vi "EEG - Independent Component Analysis.vi"() -> ()   [LabVIEW 2013]
uses:
  <vilib>/addons/Time Series Analysis/Statistical Analysis.llb/TSA Independent Component Analysis (Waveform).vi
  <vilib>/addons/Time Series Analysis/Statistical Analysis.llb/TSA Independent Component Analysis (Array).vi
  <vilib>/addons/_Advanced Signal Processing/NI_AdvSigProcTSA.lvlib
panel:
  in  "Podesavanja za metod Fast ICA":T1={"metod"=1, "maksimalna iteracija"=1000, "tolerancija konvergencije"=1e-06, "tolerancija deflacije"=1e-14, "maksimalna preciznost"=10, "tolerancija preciznosti"=1e-08} {"metod" items=["Square", "Cube", "Tanh", "Gaussian"]}
  out "Graficki prikaz rezultata":waveform(dbl)[](graph)
  out "Lokacija sacuvanog fajla na racunaru":path
  out "Signal pre analize":waveform(dbl)[](graph)
  in  "Broj nezavisnih komponenti":i32=-1
  in  "ICA metod":u16(ring) items=["Matrix Pencil ICA", "Fast ICA"]
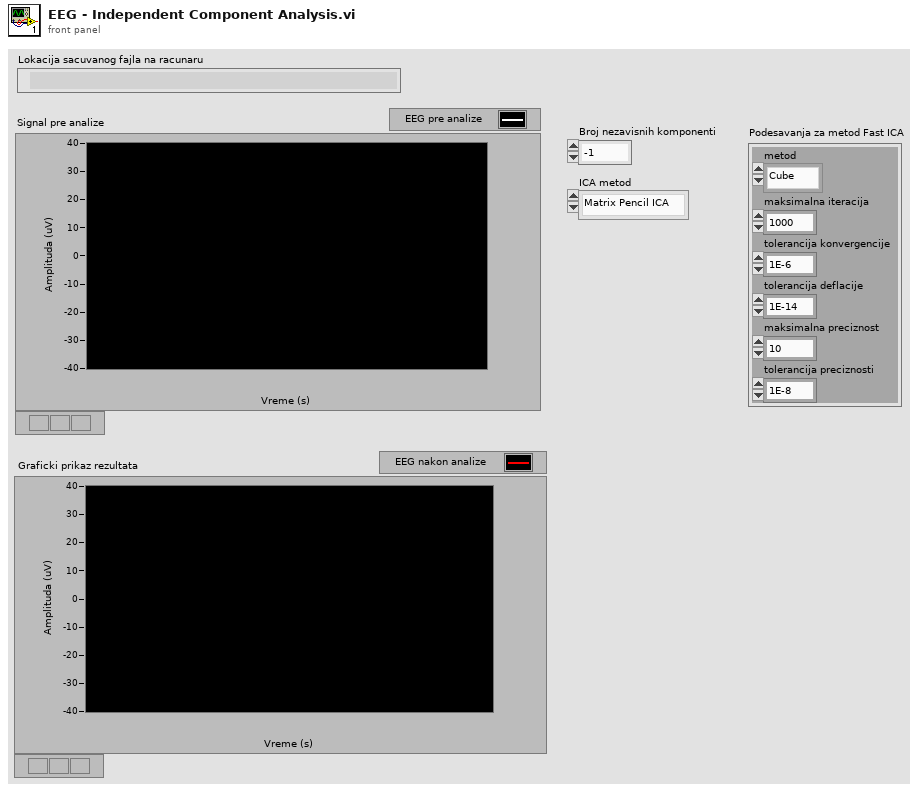
[diagram p1: front panel]
types:
  T1 = cluster{"metod":u16, "maksimalna iteracija":i32, "tolerancija konvergencije":dbl, "tolerancija deflacije":dbl, "maksimalna preciznost":i32, "tolerancija preciznosti":dbl}
  T2 = enum16{"open", "open or create", "create or replace", "create", "open (read-only)"}
  T3 = enum16{"open", "replace", "create", "open or create", "replace or create", "replace or create with confirmation"}
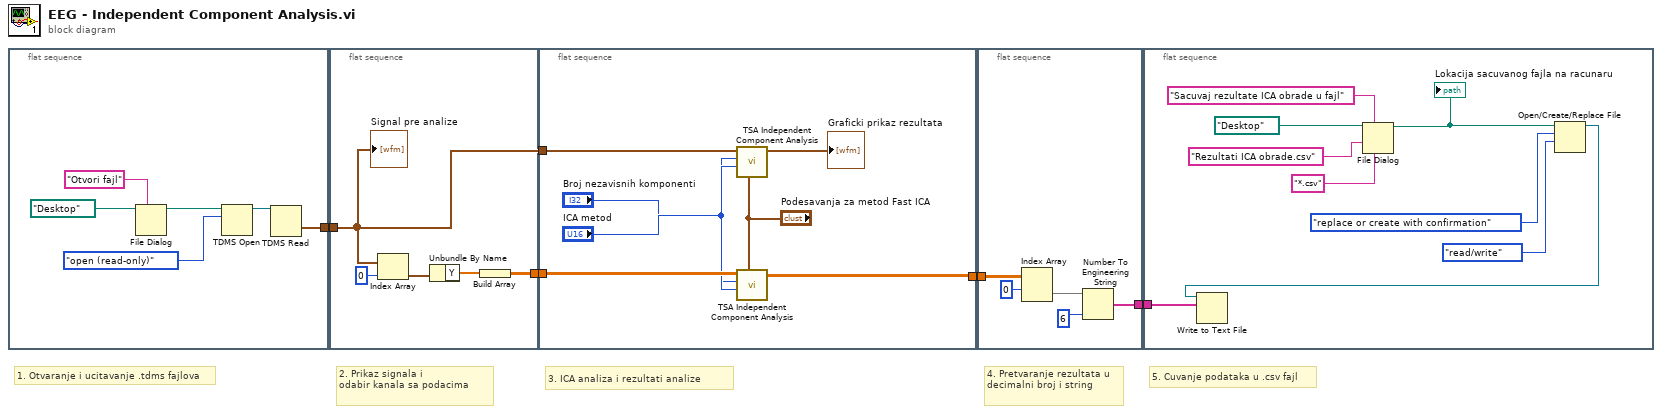
[diagram p0: block diagram]
diagram:
  # "5. Cuvanje podataka u .csv fajl"
  # "4. Pretvaranje rezultata u decimalni broj i string"
  # "3. ICA analiza i rezultati analize"
  # "2. Prikaz signala i \nodabir kanala sa podacima"
  # "1. Otvaranje i ucitavanje .tdms fajlova"
  n1 = flat-sequence {
    tunnel: [w5] -> w1
    frame #0 {
      n2 = File Dialog(7:"Otvori fajl" ("prompt"), 11:path "/Desktop" ("start path")) -> (3:w8:path)  [unwired: 2 in, 6 out]
      n3 = TDMS Open(10:T2."open (read-only)" ("operation (0:open)"), 11:w8) -> (3:w9:refnum<k34>)  [unwired: 5 in, 1 out]
      n4 = TDMS Read(0:w9) -> (10:w5:waveform(dbl)[])  [unwired: 7 in, 5 out]
    }
  }
  n5 = flat-sequence {
    tunnel: [w12] -> w2
    tunnel: w1 -> [w11]
    frame #0 {
      n6 = Index Array(array=w11, index=0) -> (element=w14:waveform(dbl))
      n7 = Unbundle By Name ("Get Waveform Components")(w14) -> ("Y"=w13:dbl[])
      n8 = Build Array(w13) -> (w12:dbl[][])
      "Signal pre analize" <- w11
    }
  }
  n9 = flat-sequence {
    tunnel: [w22] -> w3
    tunnel: w2 -> [w21]
    tunnel: w1 -> [w19]
    frame #0 {
      n10 = call-poly <vilib>:"TSA Independent Component Analysis.vi"("advanced settings"="Podesavanja za metod Fast ICA", "ICA method"="ICA metod", "number of IC"="Broj nezavisnih komponenti", "Xt"=w19) -> ("Xt out"=→"Graficki prikaz rezultata":waveform(dbl)[])  [unwired: 5 in, 2 out]
      n11 = call-poly <vilib>:"TSA Independent Component Analysis.vi"("advanced settings"="Podesavanja za metod Fast ICA", "ICA method"="ICA metod", "number of IC"="Broj nezavisnih komponenti", "Xt"=w21) -> ("Xt out"=w22:dbl[][])  [unwired: 5 in, 2 out]
    }
  }
  n12 = flat-sequence {
    tunnel: [w27] -> w4
    tunnel: w3 -> [w26]
    frame #0 {
      n13 = Index Array(array=w26, index (row)=0 ("index")) -> (element=w23:dbl[])  [unwired: 1 in]
      n14 = Number To Engineering String(2:i16 6 ("precision (6)"), 4:w23) -> (0:w27:string[])  [unwired: 2 in]
    }
  }
  n15 = flat-sequence {
    tunnel: w4 -> [w36]
    frame #0 {
      n16 = File Dialog(6:"*.csv" ("pattern (all files)"), 7:"Sacuvaj rezultate ICA obrade u fajl" ("prompt"), 9:"Rezultati ICA obrade.csv" ("default name"), 11:path "/Desktop" ("start path")) -> (3:w30:path)  [unwired: 1 in, 5 out]
      "Lokacija sacuvanog fajla na racunaru" <- w30
      n17 = Open/Create/Replace File(file path (use dialog)=w30, operation (0:open)=T3."replace or create with confirmation", access (0:read/write)=enum16{"read/write", "read-only", "write-only"}."read/write") -> (refnum out=w28:refnum<file>)  [unwired: 3 in, 2 out]
      n18 = Write to Text File(file (use dialog)=w28, text=w36) -> ()  [unwired: 2 in, 3 out]
    }
  }
